vi "Read Base.vi"(8 "error in (no error)":errorcluster, 11 "Rectangulo in":refnum<class "Rectangulo.lvclass">) -> (0 "error out":errorcluster, 2 "Base":dbl, 3 "Rectangulo out":refnum<class "Rectangulo.lvclass">)   [LabVIEW 2024, in "Rectangulo.lvclass"]
uses:
  Rectangulo.lvclass
  Rectangulo.lvclass/Rectangulo.ctl
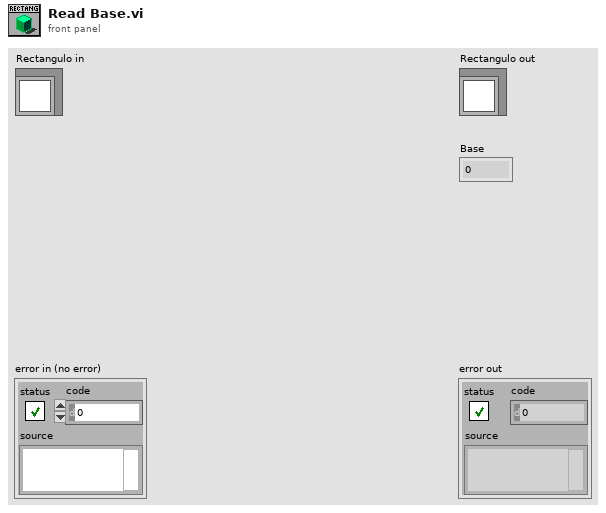
[diagram p1: front panel]
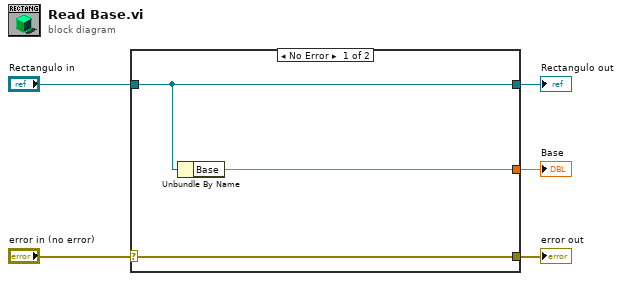
[diagram p0: block diagram]
diagram:
  n1 = case shown="No Error" "error in (no error)" {
    selector: "error in (no error)" -> [w8 w9]
    tunnel: [w8 w9] -> w4
    tunnel: [w7 w10] -> w2
    tunnel: "Rectangulo in" -> [w7 w10]
    tunnel: [w6 _] -> w1
    frame No Error {
      n2 = Unbundle By Name(w7) -> ("Base"=w6:dbl)
    }
    frame Error {
    }
  }
  "error out" <- w4
  "Rectangulo out" <- w2
  "Base" <- w1
